vi "ROI grp-Groups table menu handler.vi"(9 "ItemTag":string) -> ()   [LabVIEW 2013]
uses:
  Globals/gl_ROI grp window globals.vi
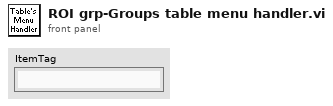
[diagram p1: front panel]
types:
  T1 = typedef "ROI grp-window ctrl refs.ctl" = cluster{"This VI":refnum<vi>, "Pane":refnum<vi>, "Table":refnum<vi>}
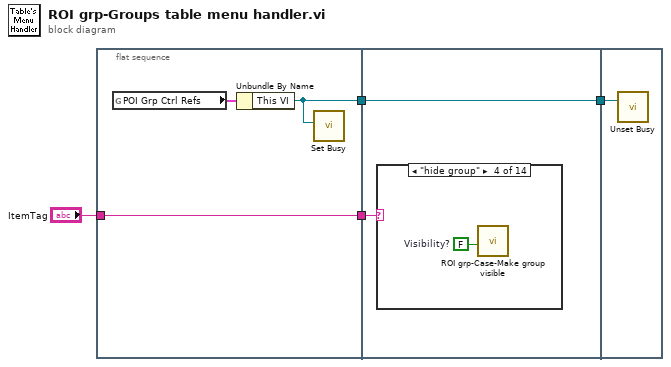
[diagram p0: block diagram]
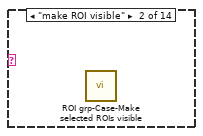
[diagram p3: hidden frame]
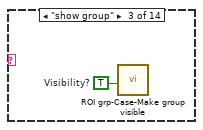
[diagram p4: hidden frame]
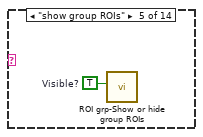
[diagram p5: hidden frame]
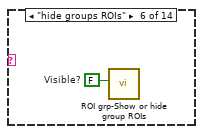
[diagram p6: hidden frame]
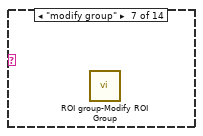
[diagram p7: hidden frame]
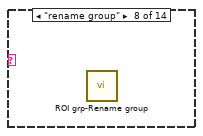
[diagram p8: hidden frame]
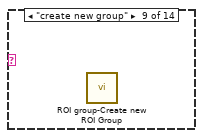
[diagram p9: hidden frame]
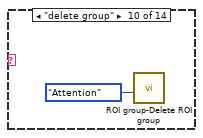
[diagram p10: hidden frame]
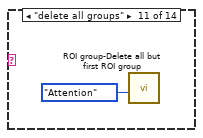
[diagram p11: hidden frame]
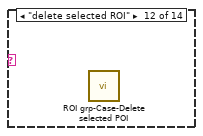
[diagram p12: hidden frame]
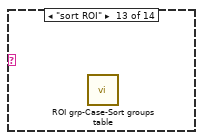
[diagram p13: hidden frame]
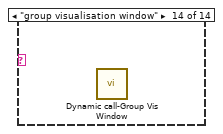
[diagram p14: hidden frame]
diagram:
  n1 = flat-sequence {
    tunnel: "ItemTag" -> [w5]
    tunnel: [w6] -> w3
    tunnel: [w5] -> w2
    tunnel: w3 -> [w9]
    tunnel: w2 -> [w8]
    tunnel: [w9] -> w1
    tunnel: w1 -> [w16]
    frame #0 {
      n2 = global read "gl_ROI grp window globals.vi" "POI Grp Ctrl Refs"() -> (w7:T1)
      n3 = Unbundle By Name(w7) -> ("This VI"=w6:refnum<vi>)
      n4 = call <vilib>:"Set Busy.vi"("VI reference (current VI)"=w6) -> ()  [unwired: 9 in, 2 out]
    }
    frame #1 {
      n5 = case shown="\"hide group\"" w8 {
        frame Default {
        }
        frame "make ROI visible" {
          n6 = call "ROI grp-Case-Make selected ROIs visible.vi"() -> ()  [unwired: 11 in, 1 out]
        }
        frame "show group" {
          w10 = TRUE  # Visibility?
          n7 = call "ROI grp-Case-Make group visible.vi"("Visibility?"=w10) -> ()  [unwired: 10 in, 1 out]
        }
        frame "hide group" {
          w11 = FALSE  # Visibility?
          n8 = call "ROI grp-Case-Make group visible.vi"("Visibility?"=w11) -> ()  [unwired: 10 in, 1 out]
        }
        frame "show group ROIs" {
          w12 = TRUE  # Visible?
          n9 = call "ROI grp-Show or hide group ROIs.vi"("Visible?"=w12) -> ()  [unwired: 10 in, 1 out]
        }
        frame "hide groups ROIs" {
          w13 = FALSE  # Visible?
          n10 = call "ROI grp-Show or hide group ROIs.vi"("Visible?"=w13) -> ()  [unwired: 10 in, 1 out]
        }
        frame "modify group" {
          n11 = call "ROI group-Modify ROI Group.vi"() -> ()  [unwired: 9 in, 3 out]
        }
        frame "rename group" {
          n12 = call "ROI grp-Rename group.vi"() -> ()  [unwired: 12 in]
        }
        frame "create new group" {
          n13 = call "ROI group-Create new ROI Group.vi"() -> ()  [unwired: 10 in, 2 out]
        }
        frame "delete group" {
          # "Deletes a group from the groups file and removes it from the control."
          n14 = call "ROI group-Delete ROI group.vi"("Dialogue message type"=enum16{"Warning", "Attention"}."Attention") -> ()  [unwired: 11 in]
        }
        frame "delete all groups" {
          # "Deletes all groups from the groups file and removes them from the control."
          n15 = call "ROI group-Delete all but first ROI group.vi"("Dialogue message type"=enum16{"Warning", "Attention"}."Attention") -> ()  [unwired: 10 in, 1 out]
        }
        frame "delete selected ROI" {
          n16 = call "ROI grp-Case-Delete selected POI.vi"() -> ()  [unwired: 11 in, 1 out]
        }
        frame "sort ROI" {
          n17 = call "ROI grp-Case-Sort groups table.vi"() -> ()  [unwired: 11 in, 1 out]
        }
        frame "group visualisation window" {
          n18 = call "Dynamic call-Group Vis Window.vi"() -> ()  [unwired: 11 in, 1 out]
        }
      }
    }
    frame #2 {
      n19 = call <vilib>:"Unset Busy.vi"("VI reference (current VI)"=w16) -> ()  [unwired: 10 in, 1 out]
    }
  }
